vi "UTF-8toGBK.vi"(9 "error in":errorcluster caption="错误输入（无错误）", 10 "UTF-8":string="测试") -> (1 "error out":errorcluster caption="错误输出", 2 "GBK":string)   [LabVIEW 2016, in "数据传输系统-05.lvlib" / "update.lvlib"]
uses:
  update.lvlib
  kernel32.dll
panel:
  out "Unicode":string
  # "\"测试\"\nUTF-8   E6B5 8BE8 AF95\nUnicode 4B6D D58B \nGBK     B2E2 CAD4"
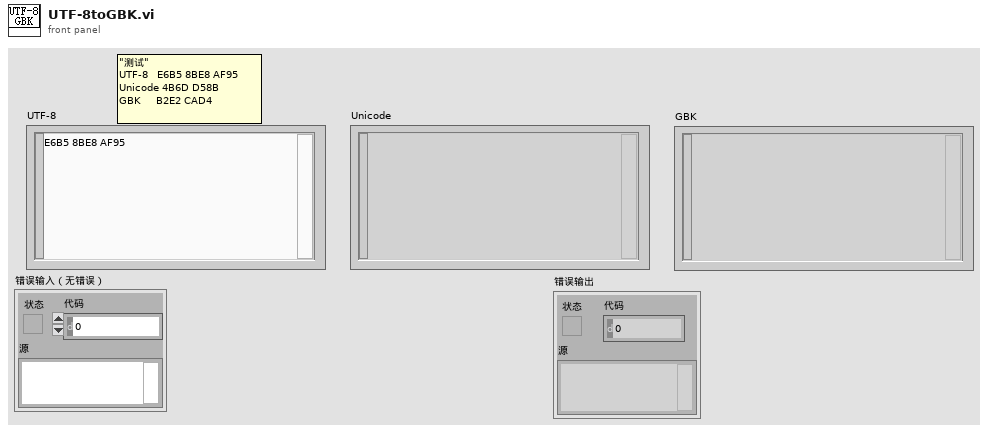
[diagram p1: front panel]
types:
  T1 = enum16{"big-endian, network order", "native, host order", "little-endian"}
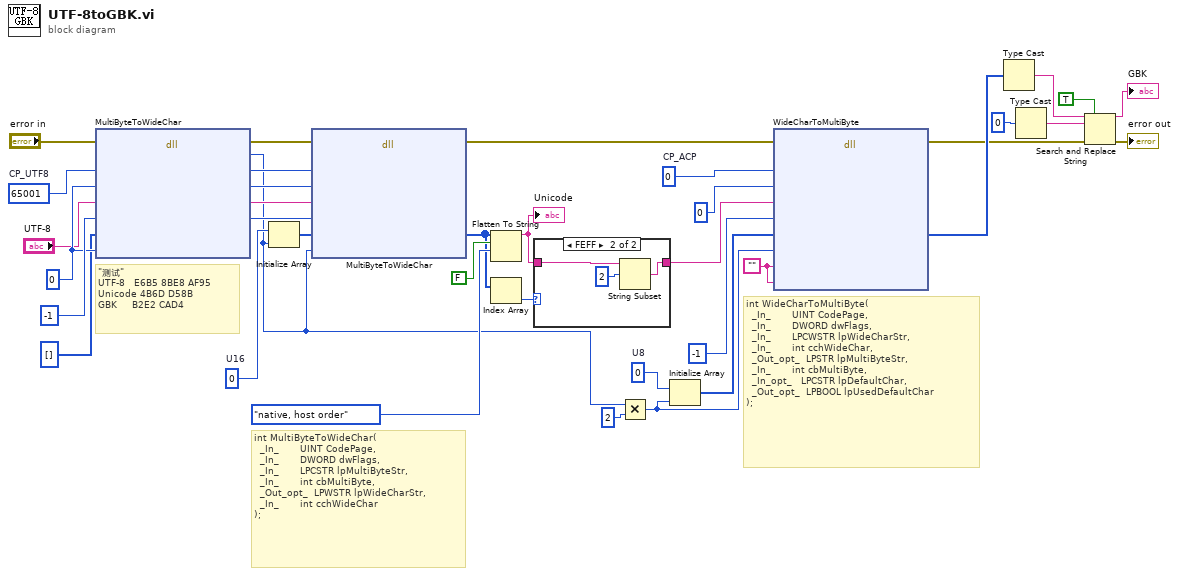
[diagram p0: block diagram]
diagram:
  w23 = u8 0  # U8
  w25 = u16 0  # U16
  w19 = u32 0  # CP_ACP
  w15 = ""
  w35 = 0 ("dwFlags")
  w34 = u32 65001  # CP_UTF8
  # "int MultiByteToWideChar(\n  _In_       UINT CodePage,\n  _In_       DWORD dwFlags,\n  _In_       LPCSTR lpMultiByteStr,\n  _In_       int cbMultiByte,\n  _Out_opt_  LPWSTR lpWideCharStr,\n  _In_       int cchWideChar\n);"
  # "int WideCharToMultiByte(\n  _In_       UINT CodePage,\n  _In_       DWORD dwFlags,\n  _In_       LPCWSTR lpWideCharStr,\n  _In_       int cchWideChar,\n  _Out_opt_  LPSTR lpMultiByteStr,\n  _In_       int cbMultiByte,\n  _In_opt_   LPCSTR lpDefaultChar,\n  _Out_opt_  LPBOOL lpUsedDefaultChar\n);"
  # "\"测试\"\nUTF-8   E6B5 8BE8 AF95\nUnicode 4B6D D58B \nGBK     B2E2 CAD4"
  n1 = dll-call lib="kernel32.dll" fn="MultiByteToWideChar"(error in="error in", "CodePage"=w34, "dwFlags"=w35, "lpMultiByteStr"="UTF-8", "cbMultiByte"=-1, "lpWideCharStr"=u16[] [], "cchWideChar"=w35) -> (error out=w37:errorcluster, "返回类型"=w12:i32, "CodePage"=w31:u32, "dwFlags"=w32:i32, "lpMultiByteStr"=w33:string, "cbMultiByte"=w30:i32)  [unwired: 4 in, 1 out]
  n2 = Initialize Array(w25, w12) -> (w24:u16[])
  n3 = dll-call lib="kernel32.dll" fn="MultiByteToWideChar"(error in=w37, "CodePage"=w31, "dwFlags"=w32, "lpMultiByteStr"=w33, "cbMultiByte"=w30, "lpWideCharStr"=w24, "cchWideChar"=w12) -> (error out=w20:errorcluster, "lpWideCharStr"=w26:u16[])  [unwired: 8 in, 1 out]
  n4 = Flatten To String(anything=w26, prepend array or string size? (T)=FALSE ("预置数组或字符串大小？(T)"), byte order (0:big-endian, network order)=T1."native, host order" ("字节顺序(0:big-endian, network order)")) -> (data string=w14:string)  [unwired: 1 in, 2 out]
  "Unicode" <- w14
  n5 = Index Array(array=w26) -> (element=w27:u16)  [unwired: 1 in]
  n6 = case shown="FEFF" w27 {
    tunnel: w14 -> [w38 w40]
    tunnel: [w38 w39] -> w17
    frame Default {
    }
    frame 65279 {
      n7 = String Subset(string=w40, offset (0)=2 ("偏移量(0)")) -> (substring=w39:string)  [unwired: 1 in]
    }
  }
  n8 = Multiply(x=w12, y=2) -> (x*y=w11:i32)
  n9 = Initialize Array(w23, w11) -> (w22:u8[])
  n10 = dll-call lib="kernel32.dll" fn="WideCharToMultiByte"(error in=w20, "CodePage"=w19, "dwFlags"=0, "lpWideCharStr"=w17, "cchWideChar"=-1, "lpMultiByteStr"=w22, "cchMultiByte"=w11, "lpDefaultChar"=w15, "pfUsedDefaultChar"=w15) -> (error out=w3:errorcluster, "lpMultiByteStr"=w10:u8[])  [unwired: 10 in, 1 out]
  n11 = Type Cast(x=w10) -> (*(type *) &x=w7:string)  [unwired: 1 in]
  n12 = Type Cast(x=u8 0 ("元素")) -> (*(type *) &x=w9:string)  [unwired: 1 in]
  n13 = Search and Replace String(replace all?=TRUE ("替换全部？(F)"), input string=w7, search string=w9, error in=w3) -> (result string=→"GBK":string, error out=→"error out":errorcluster)  [unwired: 4 in, 2 out]
